vi "SavePatientDateInfo_Hospital.vi"(8 "error in":errorcluster, 11 "hospital":T1) -> (0 "error out":errorcluster)   [LabVIEW 2013, in "main.lvlib"]
uses:
  main.lvlib
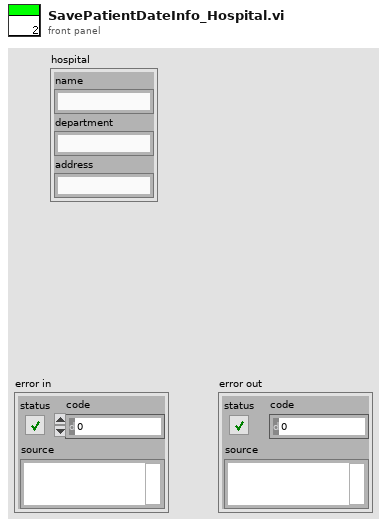
[diagram p1: front panel]
types:
  T1 = cluster{"name":string, "department":string, "address":string}
  T2 = typedef "main.lvlib/date_specific_info.ctl" = cluster{"profile":cluster{"id":string, "name":string, "operator":string, "doctor":string, "comment":string}, "hospital":cluster{"name":string, "department":string, "address":string}, "palpation":cluster{"right":string, "left":string}, "Armpressure Right":cluster{"sys":dbl, "dia":dbl, "puls":dbl, "date":string, "time":string, "code":string, "serial":string, "temp":dbl, "activity":string}[], "Armpressure Left":cluster{"sys":dbl, "dia":dbl, "puls":dbl, "date":string, "time":string, "code":string, "serial":string, "temp":dbl, "activity":string}[]}
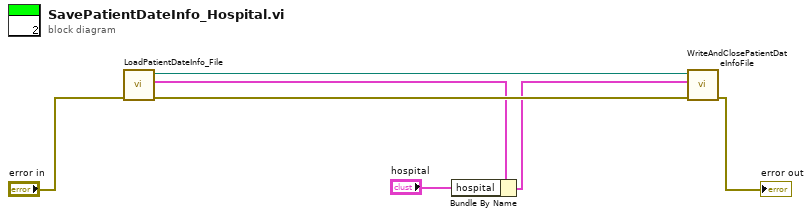
[diagram p0: block diagram]
diagram:
  n1 = call "LoadPatientDateInfo_File.vi"("error in (no error)"="error in") -> ("error out"=w6:errorcluster, "date_specific_info"=w3:T2, "path"=w5:path)  [unwired: 8 in]
  n2 = Bundle By Name(cluster=w3, "hospital"="hospital") -> (w2:T2)
  n3 = call "WriteAndClosePatientDateInfoFile.vi"("error in (no error)"=w6, "date_specific_info"=w2, "file path (use dialog)"=w5) -> ("error out"=→"error out":errorcluster)  [unwired: 8 in]
